vi "Tab Control - Set Tab Control Real Value.vi"(8 "error in (no error)":errorcluster, 9 "value":dbl, 10 "control label":string, 11 "page ref":refnum<vi>) -> (0 "error out":errorcluster)   [LabVIEW 2020]
doc: "Set real valued control by name from provided page."
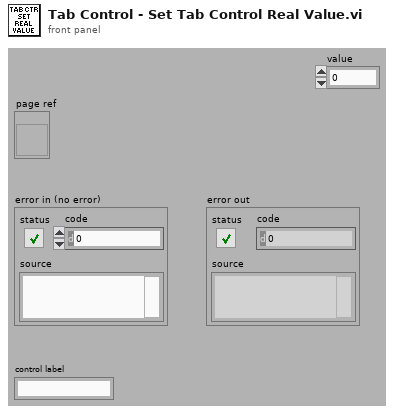
[diagram p1: front panel]
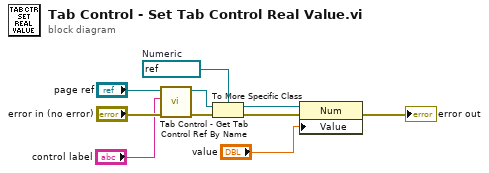
[diagram p0: block diagram]
diagram:
  w3 = refnum<vi> refnum  # Numeric
  n1 = call "Tab Control - Get Tab Control Ref By Name.vi"("error in (no error)"="error in (no error)", "control label"="control label", "page ref"="page ref") -> ("error out"=w7:errorcluster, "control ref out"=w5:refnum<vi>)  [unwired: 7 in]
  n2 = To More Specific Class(target class=w3, reference=w5, error in=w7) -> (specific class reference=w4:refnum<vi>, error out=w6:errorcluster)
  n3 = property class="Num"(reference=w4, error in=w6, "Value"="value") -> (error out=→"error out":errorcluster)  [unwired: 1 out]
